vi "Get Data Type from Path.vi"(1 "PG Path":string) -> (0 "data type":T1)   [LabVIEW 2019, in "LV-Data.PGSQL.lvclass"]
uses:
  LV-Data.PGSQL.lvclass
  Typedefs/Datatypes--enum.ctl
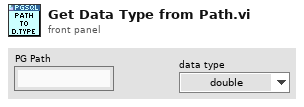
[diagram p1: front panel]
types:
  T1 = typedef "LV-Data.PGSQL.lvclass/Datatypes--enum.ctl" = enum16{"double", "string", "json", "integer", "boolean"}
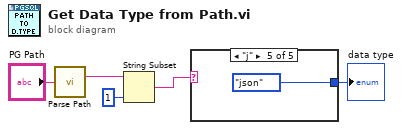
[diagram p0: block diagram]
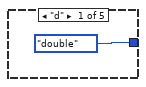
[diagram p2: hidden frame]
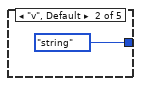
[diagram p3: hidden frame]
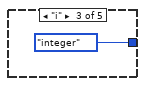
[diagram p4: hidden frame]
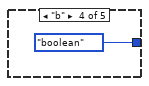
[diagram p5: hidden frame]
diagram:
  n1 = call "Parse Path.vi"("PG Path"="PG Path") -> ("Column path"=w3:string)  [unwired: 10 in, 4 out]
  n2 = String Subset(string=w3, length (rest)=1 ("length (rest)")) -> (substring=w1:string)  [unwired: 1 in]
  n3 = case shown="\"j\"" w1 {
    tunnel: [Datatypes--enum."double" ("data type") Datatypes--enum."string" ("data type") Datatypes--enum."integer" ("data type") Datatypes--enum."boolean" ("data type") Datatypes--enum."json" ("data type")] -> w4
    frame "d" {
    }
    frame "v", Default {
    }
    frame "i" {
    }
    frame "b" {
    }
    frame "j" {
    }
  }
  "data type" <- w4
